vi "OOB Update Test Cases.vi"() -> (0 "error out":errorcluster, 2 "status":string, 3 "pass":bool)   [LabVIEW 2021]
uses:
  CIFOutOfBand.lvclass/CIFOutOfBand.ctl
  CIFOutOfBand.lvclass
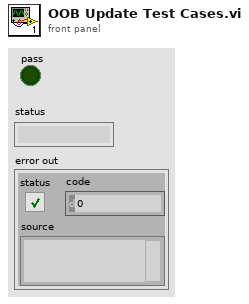
[diagram p1: front panel]
types:
  T1 = cluster{"Numeric":dbl, "Array":cluster{"Numeric":dbl, "String":string, "Boolean":bool}[], "string":string, "Null array":u8[]}
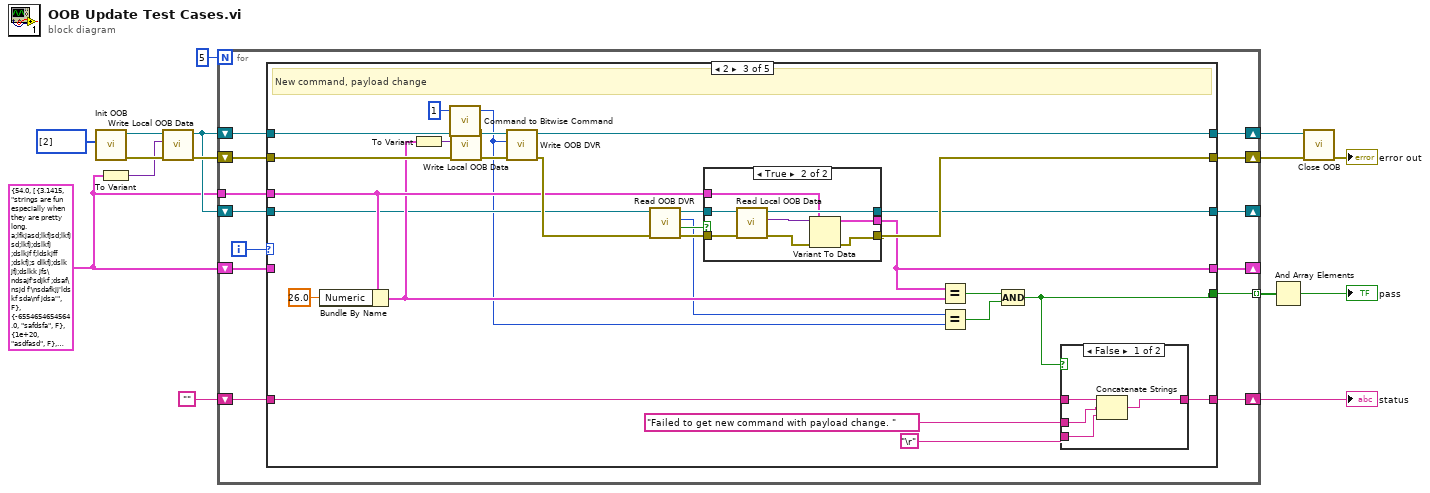
[diagram p0: block diagram]
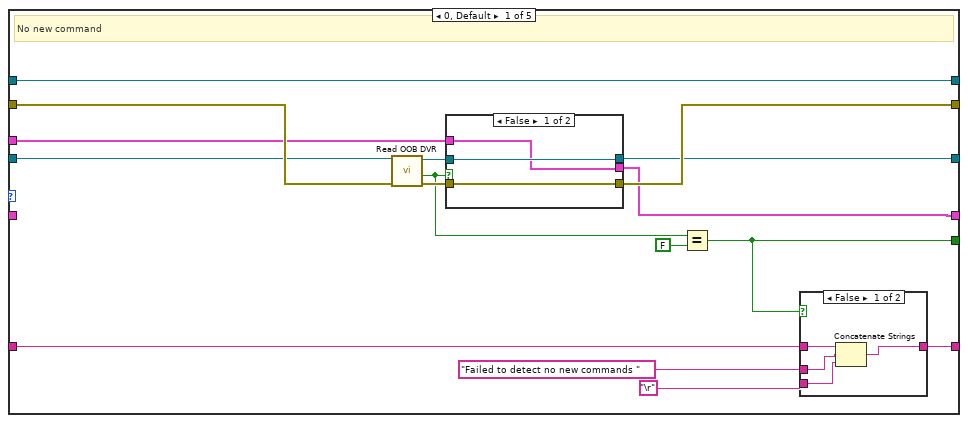
[diagram p2: hidden frame]
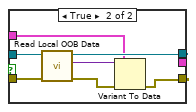
[diagram p4: hidden frame]
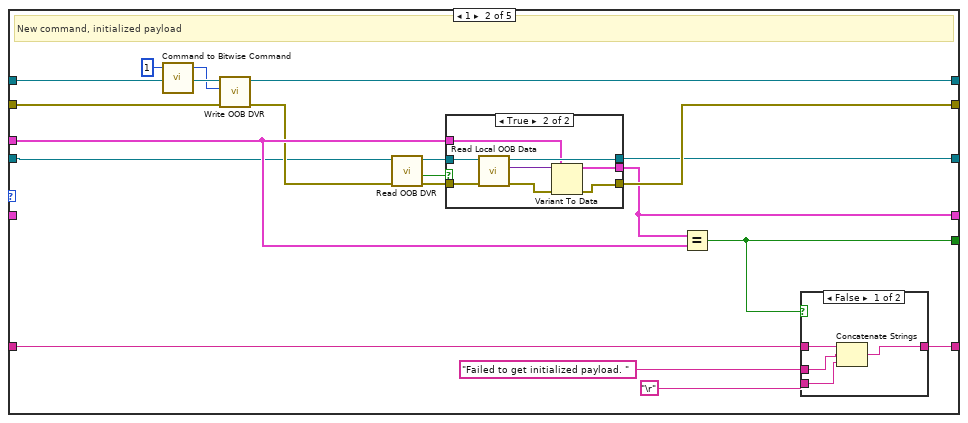
[diagram p5: hidden frame]
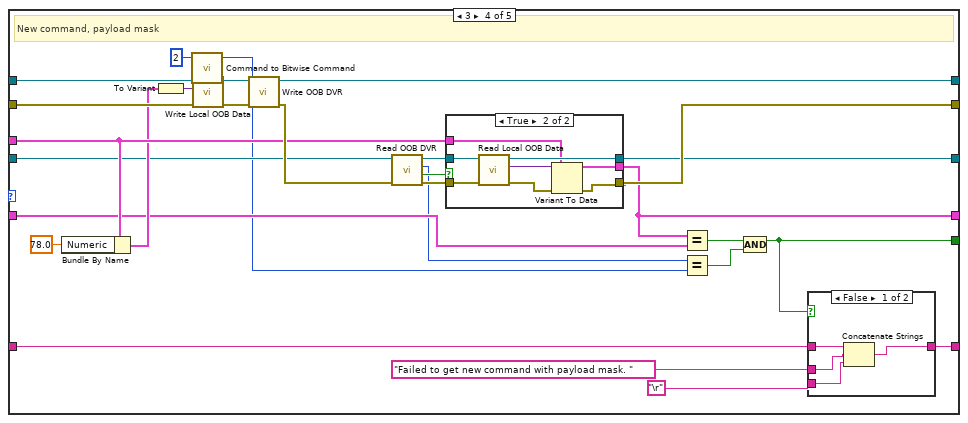
[diagram p10: hidden frame]
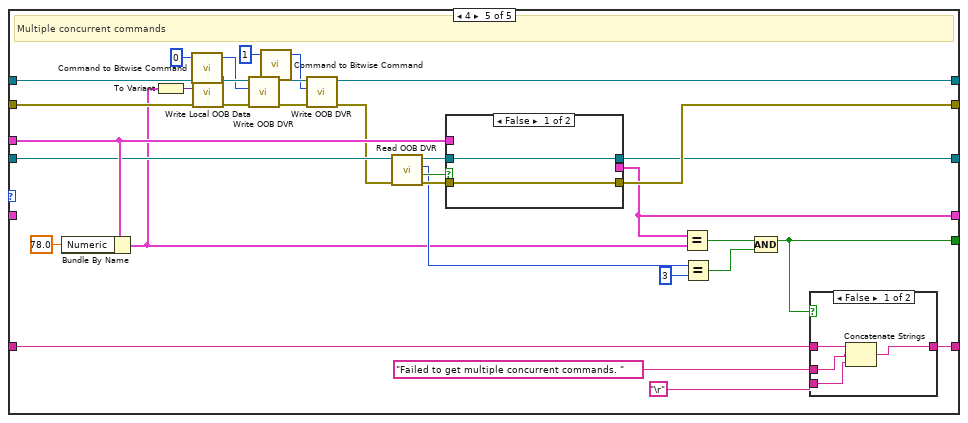
[diagram p13: hidden frame]
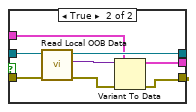
[diagram p15: hidden frame]
diagram:
  w9 = T1 {"Numeric"=54.0, "Array"=[{"Numeric"=3.1415, "String"="strings are fun especially when they are pretty long. a;lfkjasd;lkfjsd;lkfjsd;lkfj;dslkfj ;dslkjf f;ldskjff ;dskfj;s dlkfj;dslk jfj;dslkk jfs\ndsajf'sdjkf ;dsaf\nsjd f'\nsdafkjj'lds kf sda\nf jdsa'", "Boolean"=FALSE}, {"Numeric"=-6554654654564.0, "String"="safdsfa", "Boolean"=FALSE}, {"Numeric"=1e+20, "String"="asdfasd", "Boolean"=FALSE}, {"Numeric"=2.0, "String"="afd", "Boolean"=TRUE}, {"Numeric"=12.34, "String"="data", "Boolean"=FALSE}], "string"="strings", "Null array"=[0]} ("Test Config")
  n1 = call "Init OOB.vi"("Cases to Skip Payload"=u8[] [2]) -> ("error out"=w15:errorcluster, "OOB out"=w13:refnum<class "CIFOutOfBand.lvclass">)  [unwired: 9 in]
  n2 = To Variant(anything=w9) -> (Variant=w14:variant)
  n3 = call "Write Local OOB Data.vi"("error in"=w15, "Local OOB Data"=w14, "OOB in"=w13) -> ("error out"=w12:errorcluster, "OOB out"=w11:refnum<class "CIFOutOfBand.lvclass">)  [unwired: 7 in]
  n4 = for {
    N: 5 -> [_]
    tunnel: [w28] -> w6 mode=indexing
    tunnel: w9 -> [w26]
    shift-right: [w24] -> w7
    shift-left: w12 -> [w27]
    shift-right: [w22] -> w8
    shift-left: w11 -> [w25]
    shift-right: [w20] -> _
    shift-left: w11 -> [w21]
    shift-right: [w19] -> _
    shift-left: w9 -> [w18]
    shift-right: [w16] -> w1
    shift-left: "" -> [w17]
    i -> [w23]
    n5 = case shown="2" w23 {
      tunnel: [w35 w61 w94 w137 w179] -> w28
      tunnel: w27 -> [w42 w72 w113 w156 w204]
      tunnel: w26 -> [w41 w75 w108 w151 w199]
      tunnel: w25 -> [w38 w73 w114 w157 w205]
      tunnel: [w40 w74 w117 w160 w207] -> w24
      tunnel: [w38 w68 w106 w149 w189] -> w22
      tunnel: w21 -> [w37 w66 w105 w148 w198]
      tunnel: [w39 w67 w104 w147 w197] -> w20
      tunnel: [w36 w65 w103 w145 w196] -> w19
      tunnel: w18 -> [_ _ _ w146 _]
      tunnel: w17 -> [w34 w60 w96 w138 w180]
      tunnel: [w33 w62 w95 w136 w181] -> w16
      frame 0, Default {
        # "No new command"
        n6 = call "Read OOB DVR.vi"("error in"=w42, "OOB in"=w37) -> ("error out"=w43:errorcluster, "New Commands"=w32:bool, "OOB out"=w44:refnum<class "CIFOutOfBand.lvclass">)  [unwired: 6 in, 1 out]
        n7 = case shown="False" w32 {
          tunnel: w44 -> [w51 w59]
          tunnel: w43 -> [w52 w58]
          tunnel: [w51 w56] -> w39
          tunnel: w41 -> [w50 w54]
          tunnel: [w50 _] -> w36
          tunnel: [w52 w53] -> w40
          frame False {
          }
          frame True {
            n8 = call "Read Local OOB Data.vi"("error in"=w58, "OOB in"=w59) -> ("error out"=w57:errorcluster, "Local OOB Data"=w55:variant, "OOB out"=w56:refnum<class "CIFOutOfBand.lvclass">)  [unwired: 7 in]
            n9 = Variant To Data(error in=w57, type=w54, Variant=w55) -> (error out=w53:errorcluster)  [unwired: 1 out]
          }
        }
        n10 = Equal?(x=w32, y=FALSE) -> (x = y?=w35:bool)
        n11 = case shown="False" w35 {
          tunnel: w34 -> [w48 w49]
          tunnel: [w45 w49] -> w33
          tunnel: "Failed to detect no new commands " -> [w47 _]
          tunnel: "\r" -> [w46 _]
          frame False {
            n12 = Concatenate Strings(w48, w47, w46) -> (w45:string)
          }
          frame True {
          }
        }
      }
      frame 1 {
        # "New command, initialized payload"
        n13 = call "Command to Bitwise Command.vi"("OOB Command"=u8 1) -> ("bit command"=w70:u64)  [unwired: 3 in]
        n14 = call "Write OOB DVR.vi"("error in"=w72, "Commands (bitwise)"=w70, "OOB in"=w73) -> ("error out"=w71:errorcluster, "OOB out"=w68:refnum<class "CIFOutOfBand.lvclass">)  [unwired: 7 in]
        n15 = call "Read OOB DVR.vi"("error in"=w71, "OOB in"=w66) -> ("error out"=w76:errorcluster, "New Commands"=w78:bool, "OOB out"=w77:refnum<class "CIFOutOfBand.lvclass">)  [unwired: 6 in, 1 out]
        n16 = case shown="True" w78 {
          tunnel: w77 -> [w84 w93]
          tunnel: w76 -> [w85 w92]
          tunnel: [w84 w90] -> w67
          tunnel: w75 -> [_ w88]
          tunnel: [_ w86] -> w65
          tunnel: [w85 w87] -> w74
          frame False {
          }
          frame True {
            n17 = call "Read Local OOB Data.vi"("error in"=w92, "OOB in"=w93) -> ("error out"=w91:errorcluster, "Local OOB Data"=w89:variant, "OOB out"=w90:refnum<class "CIFOutOfBand.lvclass">)  [unwired: 7 in]
            n18 = Variant To Data(error in=w91, type=w88, Variant=w89) -> (data=w86:T1, error out=w87:errorcluster)
          }
        }
        n19 = Equal?(x=w65, y=w75) -> (x = y?=w61:bool)
        n20 = case shown="False" w61 {
          tunnel: w60 -> [w82 w83]
          tunnel: [w79 w83] -> w62
          tunnel: "Failed to get initialized payload. " -> [w81 _]
          tunnel: "\r" -> [w80 _]
          frame False {
            n21 = Concatenate Strings(w82, w81, w80) -> (w79:string)
          }
          frame True {
          }
        }
      }
      frame 2 {
        # "New command, payload change"
        n22 = Bundle By Name(cluster=w108, "Numeric"=26.0) -> (w107:T1)
        n23 = To Variant(anything=w107) -> (Variant=w109:variant)
        n24 = call "Command to Bitwise Command.vi"("OOB Command"=u8 1) -> ("bit command"=w99:u64)  [unwired: 3 in]
        n25 = call "Write Local OOB Data.vi"("error in"=w113, "Local OOB Data"=w109, "OOB in"=w114) -> ("error out"=w111:errorcluster, "OOB out"=w112:refnum<class "CIFOutOfBand.lvclass">)  [unwired: 7 in]
        n26 = call "Write OOB DVR.vi"("error in"=w111, "Commands (bitwise)"=w99, "OOB in"=w112) -> ("error out"=w116:errorcluster, "OOB out"=w106:refnum<class "CIFOutOfBand.lvclass">)  [unwired: 7 in]
        n27 = call "Read OOB DVR.vi"("error in"=w116, "OOB in"=w105) -> ("error out"=w118:errorcluster, "New Commands"=w120:bool, "Commands (bitwise)"=w100:u64, "OOB out"=w119:refnum<class "CIFOutOfBand.lvclass">)  [unwired: 6 in]
        n28 = case shown="True" w120 {
          tunnel: w119 -> [w126 w135]
          tunnel: w118 -> [w127 w134]
          tunnel: [w126 w132] -> w104
          tunnel: w108 -> [_ w130]
          tunnel: [_ w128] -> w103
          tunnel: [w127 w129] -> w117
          frame False {
          }
          frame True {
            n29 = call "Read Local OOB Data.vi"("error in"=w134, "OOB in"=w135) -> ("error out"=w133:errorcluster, "Local OOB Data"=w131:variant, "OOB out"=w132:refnum<class "CIFOutOfBand.lvclass">)  [unwired: 7 in]
            n30 = Variant To Data(error in=w133, type=w130, Variant=w131) -> (data=w128:T1, error out=w129:errorcluster)
          }
        }
        n31 = Equal?(x=w103, y=w107) -> (x = y?=w102:bool)
        n32 = Equal?(x=w100, y=w99) -> (x = y?=w101:bool)
        n33 = Compound Arithmetic op=AND(w102, w101) -> (w94:bool)
        n34 = case shown="False" w94 {
          tunnel: w96 -> [w124 w125]
          tunnel: [w121 w125] -> w95
          tunnel: "Failed to get new command with payload change. " -> [w123 _]
          tunnel: "\r" -> [w122 _]
          frame False {
            n35 = Concatenate Strings(w124, w123, w122) -> (w121:string)
          }
          frame True {
          }
        }
      }
      frame 3 {
        # "New command, payload mask"
        n36 = Bundle By Name(cluster=w151, "Numeric"=78.0) -> (w150:T1)
        n37 = To Variant(anything=w150) -> (Variant=w152:variant)
        n38 = call "Command to Bitwise Command.vi"("OOB Command"=u8 2) -> ("bit command"=w142:u64)  [unwired: 3 in]
        n39 = call "Write Local OOB Data.vi"("error in"=w156, "Local OOB Data"=w152, "OOB in"=w157) -> ("error out"=w154:errorcluster, "OOB out"=w155:refnum<class "CIFOutOfBand.lvclass">)  [unwired: 7 in]
        n40 = call "Write OOB DVR.vi"("error in"=w154, "Commands (bitwise)"=w142, "OOB in"=w155) -> ("error out"=w159:errorcluster, "OOB out"=w149:refnum<class "CIFOutOfBand.lvclass">)  [unwired: 7 in]
        n41 = call "Read OOB DVR.vi"("error in"=w159, "OOB in"=w148) -> ("error out"=w161:errorcluster, "New Commands"=w163:bool, "Commands (bitwise)"=w143:u64, "OOB out"=w162:refnum<class "CIFOutOfBand.lvclass">)  [unwired: 6 in]
        n42 = case shown="True" w163 {
          tunnel: w162 -> [w169 w178]
          tunnel: w161 -> [w170 w177]
          tunnel: [w169 w175] -> w147
          tunnel: w151 -> [_ w173]
          tunnel: [_ w171] -> w145
          tunnel: [w170 w172] -> w160
          frame False {
          }
          frame True {
            n43 = call "Read Local OOB Data.vi"("error in"=w177, "OOB in"=w178) -> ("error out"=w176:errorcluster, "Local OOB Data"=w174:variant, "OOB out"=w175:refnum<class "CIFOutOfBand.lvclass">)  [unwired: 7 in]
            n44 = Variant To Data(error in=w176, type=w173, Variant=w174) -> (data=w171:T1, error out=w172:errorcluster)
          }
        }
        n45 = Equal?(x=w145, y=w146) -> (x = y?=w144:bool)
        n46 = Equal?(x=w143, y=w142) -> (x = y?=w141:bool)
        n47 = Compound Arithmetic op=AND(w144, w141) -> (w137:bool)
        n48 = case shown="False" w137 {
          tunnel: w138 -> [w167 w168]
          tunnel: [w164 w168] -> w136
          tunnel: "Failed to get new command with payload mask. " -> [w166 _]
          tunnel: "\r" -> [w165 _]
          frame False {
            n49 = Concatenate Strings(w167, w166, w165) -> (w164:string)
          }
          frame True {
          }
        }
      }
      frame 4 {
        # "Multiple concurrent commands"
        n50 = Bundle By Name(cluster=w199, "Numeric"=78.0) -> (w184:T1)
        n51 = To Variant(anything=w184) -> (Variant=w200:variant)
        n52 = call "Command to Bitwise Command.vi"("OOB Command"=u8 0) -> ("bit command"=w193:u64)  [unwired: 3 in]
        n53 = call "Write Local OOB Data.vi"("error in"=w204, "Local OOB Data"=w200, "OOB in"=w205) -> ("error out"=w202:errorcluster, "OOB out"=w203:refnum<class "CIFOutOfBand.lvclass">)  [unwired: 7 in]
        n54 = call "Write OOB DVR.vi"("error in"=w202, "Commands (bitwise)"=w193, "OOB in"=w203) -> ("error out"=w191:errorcluster, "OOB out"=w190:refnum<class "CIFOutOfBand.lvclass">)  [unwired: 7 in]
        n55 = call "Command to Bitwise Command.vi"("OOB Command"=u8 1) -> ("bit command"=w188:u64)  [unwired: 3 in]
        n56 = call "Write OOB DVR.vi"("error in"=w191, "Commands (bitwise)"=w188, "OOB in"=w190) -> ("error out"=w186:errorcluster, "OOB out"=w189:refnum<class "CIFOutOfBand.lvclass">)  [unwired: 7 in]
        n57 = call "Read OOB DVR.vi"("error in"=w186, "OOB in"=w198) -> ("error out"=w208:errorcluster, "New Commands"=w210:bool, "Commands (bitwise)"=w194:u64, "OOB out"=w209:refnum<class "CIFOutOfBand.lvclass">)  [unwired: 6 in]
        n58 = case shown="False" w210 {
          tunnel: w209 -> [w216 w225]
          tunnel: w208 -> [w217 w224]
          tunnel: [w216 w222] -> w197
          tunnel: w199 -> [_ w220]
          tunnel: [_ w218] -> w196
          tunnel: [w217 w219] -> w207
          frame False {
          }
          frame True {
            n59 = call "Read Local OOB Data.vi"("error in"=w224, "OOB in"=w225) -> ("error out"=w223:errorcluster, "Local OOB Data"=w221:variant, "OOB out"=w222:refnum<class "CIFOutOfBand.lvclass">)  [unwired: 7 in]
            n60 = Variant To Data(error in=w223, type=w220, Variant=w221) -> (data=w218:T1, error out=w219:errorcluster)
          }
        }
        n61 = Equal?(x=w196, y=w184) -> (x = y?=w195:bool)
        n62 = Equal?(x=w194, y=u64 3) -> (x = y?=w192:bool)
        n63 = Compound Arithmetic op=AND(w195, w192) -> (w179:bool)
        n64 = case shown="False" w179 {
          tunnel: w180 -> [w214 w215]
          tunnel: [w211 w215] -> w181
          tunnel: "Failed to get multiple concurrent commands. " -> [w213 _]
          tunnel: "\r" -> [w212 _]
          frame False {
            n65 = Concatenate Strings(w214, w213, w212) -> (w211:string)
          }
          frame True {
          }
        }
      }
    }
  }
  "status" <- w1
  n66 = And Array Elements(Boolean array=w6) -> (logical AND=→"pass":bool)
  n67 = call "Close OOB.vi"("error in"=w7, "OOB in"=w8) -> ("error out"=→"error out":errorcluster)  [unwired: 9 in]
